vi "Display Parameter Switch.vi"(10 "L_Or_R":string, 11 "Switch":T2(ring)) -> (1 "State":T1, 2 "Data Path":string[](array[string]), 3 "Column":string[](array[string]))   [LabVIEW 2015, in "Utility VIs.lvlib"]
uses:
  Utility VIs.lvlib
  Sample/Support/Result Panel State.ctl
  Sample/Sample.lvlib
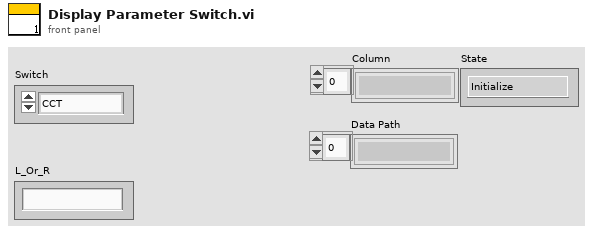
[diagram p1: front panel]
types:
  T1 = typedef "Sample.lvlib/Result Panel State.ctl" = enum16{"Initialize", "Connect Database", "Select Database", "Register", "Wait For Event", "Start", "Calculation", "Display Result", "OS Summary Update", "OS Parameter List Update", "OD Summary Update", "OD Parameter List Update", "Exit", "OD IMG Parameter List Update", "OS IMG Parameter List Update"}
  T2 = enum16{"CCT", "ACD", "LT", "RT", "AL", "PD", "WTW", "K_flat", "K_steep", "K_AST"}
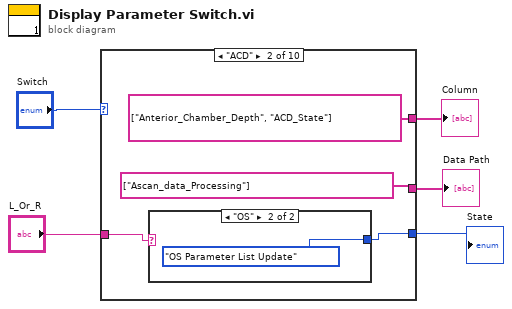
[diagram p0: block diagram]
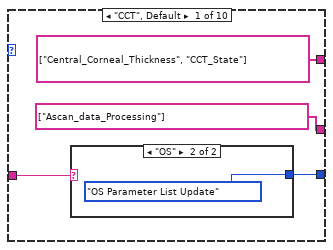
[diagram p2: hidden frame]
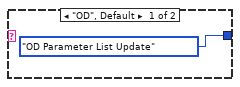
[diagram p3: hidden frame]
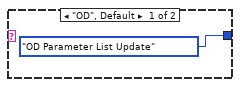
[diagram p4: hidden frame]
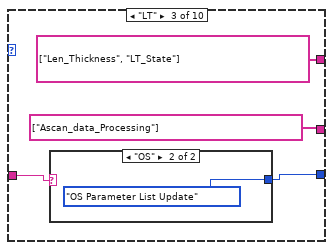
[diagram p5: hidden frame]
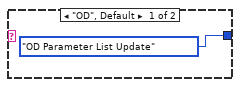
[diagram p6: hidden frame]
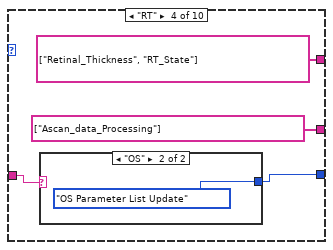
[diagram p7: hidden frame]
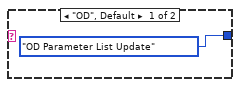
[diagram p8: hidden frame]
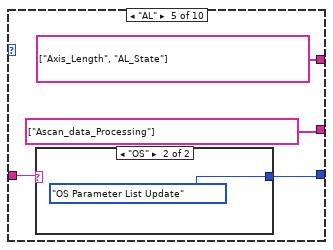
[diagram p9: hidden frame]
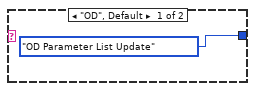
[diagram p10: hidden frame]
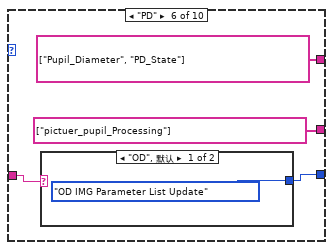
[diagram p11: hidden frame]
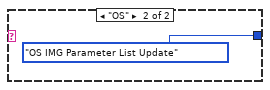
[diagram p12: hidden frame]
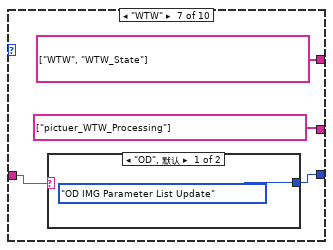
[diagram p13: hidden frame]
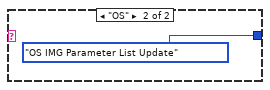
[diagram p14: hidden frame]
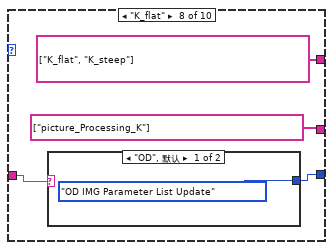
[diagram p15: hidden frame]
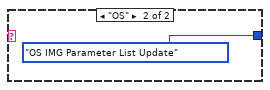
[diagram p16: hidden frame]
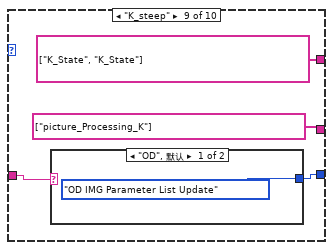
[diagram p17: hidden frame]
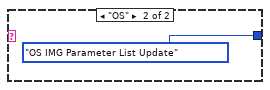
[diagram p18: hidden frame]
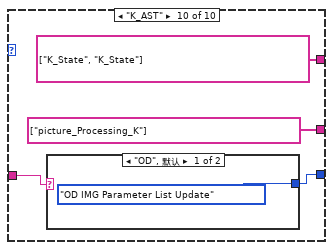
[diagram p19: hidden frame]
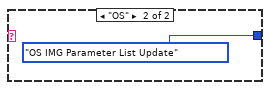
[diagram p20: hidden frame]
diagram:
  n1 = case shown="\"ACD\"" "Switch" {
    tunnel: [string[] ["Central_Corneal_Thickness", "CCT_State"] string[] ["Anterior_Chamber_Depth", "ACD_State"] string[] ["Len_Thickness", "LT_State"] string[] ["Retinal_Thickness", "RT_State"] string[] ["Axis_Length", "AL_State"] string[] ["Pupil_Diameter", "PD_State"] string[] ["WTW", "WTW_State"] string[] ["K_flat", "K_steep"] string[] ["K_State", "K_State"] string[] ["K_State", "K_State"]] -> w4
    tunnel: [string[] ["Ascan_data_Processing"] string[] ["Ascan_data_Processing"] string[] ["Ascan_data_Processing"] string[] ["Ascan_data_Processing"] string[] ["Ascan_data_Processing"] string[] ["pictuer_pupil_Processing"] string[] ["pictuer_WTW_Processing"] string[] ["picture_Processing_K"] string[] ["picture_Processing_K"] string[] ["picture_Processing_K"]] -> w3
    tunnel: [w7 w12 w18 w24 w30 w36 w42 w48 w54 w60] -> w2
    tunnel: "L_Or_R" -> [w6 w13 w19 w25 w31 w37 w43 w49 w55 w61]
    frame "CCT", Default {
      n2 = case shown="\"OS\"" w6 {
        tunnel: [Result_Panel_State."OD Parameter List Update" ("State") Result_Panel_State."OS Parameter List Update" ("State")] -> w7
        frame "OD", Default {
        }
        frame "OS" {
        }
      }
    }
    frame "ACD" {
      n3 = case shown="\"OS\"" w13 {
        tunnel: [Result_Panel_State."OD Parameter List Update" ("State") Result_Panel_State."OS Parameter List Update" ("State")] -> w12
        frame "OD", Default {
        }
        frame "OS" {
        }
      }
    }
    frame "LT" {
      n4 = case shown="\"OS\"" w19 {
        tunnel: [Result_Panel_State."OD Parameter List Update" ("State") Result_Panel_State."OS Parameter List Update" ("State")] -> w18
        frame "OD", Default {
        }
        frame "OS" {
        }
      }
    }
    frame "RT" {
      n5 = case shown="\"OS\"" w25 {
        tunnel: [Result_Panel_State."OD Parameter List Update" ("State") Result_Panel_State."OS Parameter List Update" ("State")] -> w24
        frame "OD", Default {
        }
        frame "OS" {
        }
      }
    }
    frame "AL" {
      n6 = case shown="\"OS\"" w31 {
        tunnel: [Result_Panel_State."OD Parameter List Update" ("State") Result_Panel_State."OS Parameter List Update" ("State")] -> w30
        frame "OD", Default {
        }
        frame "OS" {
        }
      }
    }
    frame "PD" {
      n7 = case shown="\"OD\", 默认" w37 {
        tunnel: [Result_Panel_State."OD IMG Parameter List Update" ("State") Result_Panel_State."OS IMG Parameter List Update" ("State")] -> w36
        frame "OD", Default {
        }
        frame "OS" {
        }
      }
    }
    frame "WTW" {
      n8 = case shown="\"OD\", 默认" w43 {
        tunnel: [Result_Panel_State."OD IMG Parameter List Update" ("State") Result_Panel_State."OS IMG Parameter List Update" ("State")] -> w42
        frame "OD", Default {
        }
        frame "OS" {
        }
      }
    }
    frame "K_flat" {
      n9 = case shown="\"OD\", 默认" w49 {
        tunnel: [Result_Panel_State."OD IMG Parameter List Update" ("State") Result_Panel_State."OS IMG Parameter List Update" ("State")] -> w48
        frame "OD", Default {
        }
        frame "OS" {
        }
      }
    }
    frame "K_steep" {
      n10 = case shown="\"OD\", 默认" w55 {
        tunnel: [Result_Panel_State."OD IMG Parameter List Update" ("State") Result_Panel_State."OS IMG Parameter List Update" ("State")] -> w54
        frame "OD", Default {
        }
        frame "OS" {
        }
      }
    }
    frame "K_AST" {
      n11 = case shown="\"OD\", 默认" w61 {
        tunnel: [Result_Panel_State."OD IMG Parameter List Update" ("State") Result_Panel_State."OS IMG Parameter List Update" ("State")] -> w60
        frame "OD", Default {
        }
        frame "OS" {
        }
      }
    }
  }
  "Column" <- w4
  "Data Path" <- w3
  "State" <- w2
